vi "Provider_OnPopupMenu.vi"(11 "objects":T1[](array[typedef])) -> ()   [LabVIEW 2020, in "Actor Message Maker Provider.lvlib"]
uses:
  Actor Message Maker Provider.lvlib
  <resource>/Framework/Providers/API/mxLvMenuItem.ctl
  MessageMakerProvider/Support/Localized Strings.vi
  MessageMakerProvider/Message Maker Provider.lvlib
  MessageMakerProvider/AFPP Shared/Validation Mode.ctl
  MessageMakerProvider/AFPP Shared/AFPP Shared.lvlib
  <resource>/Framework/Providers/API/ItemRef.ctl
panel:
  out "error out":errorcluster
  in  "error in":errorcluster
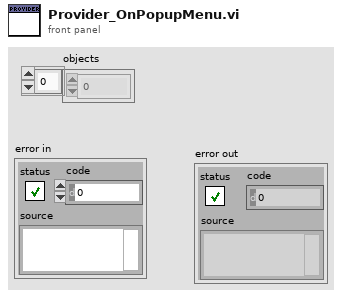
[diagram p1: front panel]
types:
  T1 = typedef "ItemRef.ctl" = u64
  T2 = typedef "AFPP Shared.lvlib/Validation Mode.ctl" = enum16{"An Actor Library", "A Target Tag"}
  T3 = typedef "mxLvMenuItem.ctl" = cluster{"Menu Name":string, "Description":string, "Icon File Name":path, "Menu Tag":string, "Enabled":bool, "Checked":bool, "Separator":bool, "Batchable":bool, "Weight":i32, "Batch Mode (Ignored if Not Batchable)":enum32{"Show If All Items Support Command", "Show If Any Items Support Command"}, "Menu Location":enum32{"<None>", "Project", "Project / Build Specifications", "Tools", "Tools / Source Control", "Tools / Real-Time Module", "Help"}, "Exclude From Getting Started Window Menu":bool}
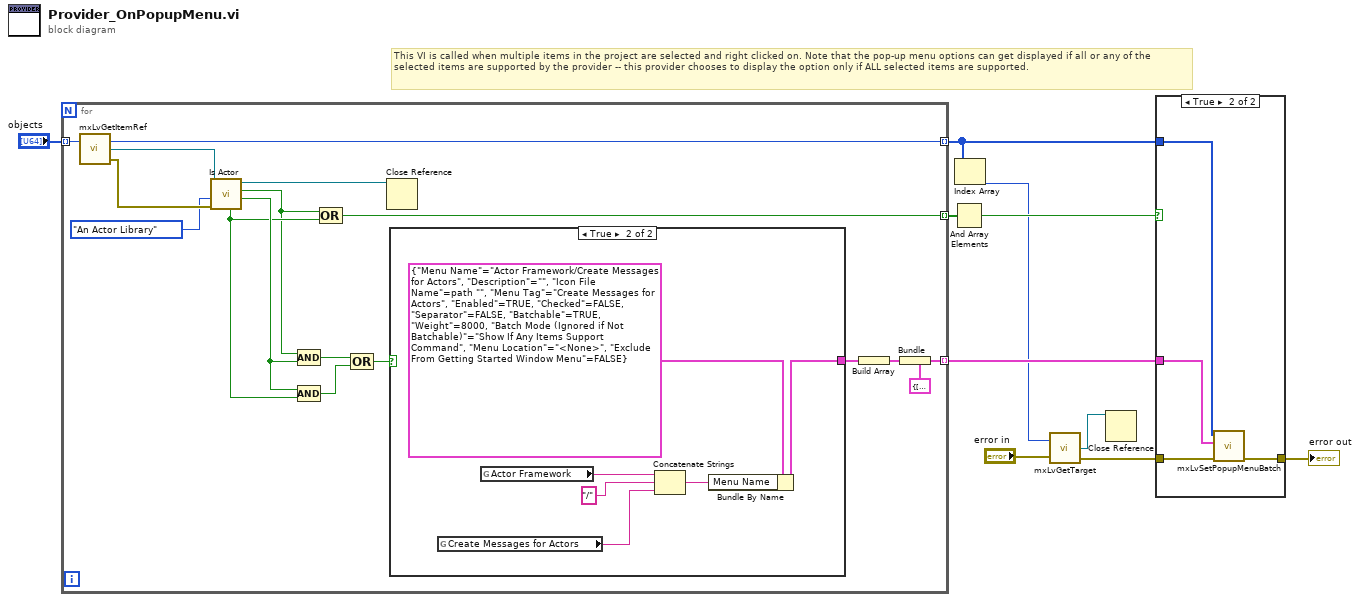
[diagram p0: block diagram]
diagram:
  # "This VI is called when multiple items in the project are selected and right clicked on. Note that the pop-up menu options can get displayed if all or any of the selected items are supported by the provider -- this provider chooses to display the option only if ALL selected items are supported."
  n1 = for {
    tunnel: [w27] -> w10 mode=indexing
    tunnel: "objects" -> [w26] mode=indexing
    tunnel: [w25] -> w2 mode=indexing
    tunnel: [w11] -> w7 mode=indexing
    n2 = call <resource>:"mxLvGetItemRef.vi"("Item"=w26) -> ("Item"=w25:T1, "Item Refnum"=w22:refnum<vi>, "error out"=w21:errorcluster)  [unwired: 1 in]
    n3 = call "Is Actor.vi"("error in (no error)"=w21, "Validation"=Validation_Mode."An Actor Library", "ProjectItem in"=w22) -> ("Has Public Methods"=w15:bool, "Is Actor"=w12:bool, "ProjectItem out"=w23:refnum<vi>, "Is Actor Interface"=w13:bool)  [unwired: 4 in, 1 out]
    n4 = Compound Arithmetic op=AND(w12, w15) -> (w16:bool)
    n5 = Compound Arithmetic op=AND(w15, w13) -> (w14:bool)
    n6 = Compound Arithmetic op=OR(w12, w13) -> (w11:bool)
    n7 = Compound Arithmetic op=OR(w16, w14) -> (w17:bool)
    n8 = Close Reference(reference=w23) -> ()  [unwired: 1 in, 1 out]
    n9 = case shown="True" w17 {
      tunnel: [_ w32] -> w20
      frame False {
      }
      frame True {
        n10 = global read "Localized Strings.vi" "Create Messages for Actors"() -> (w28:string)
        n11 = global read "Localized Strings.vi" "Actor Framework"() -> (w31:string)
        n12 = Concatenate Strings(w31, "/", w28) -> (w29:string)
        n13 = Bundle By Name(cluster=T3 {"Menu Name"="Actor Framework/Create Messages for Actors", "Description"="", "Icon File Name"=path "", "Menu Tag"="Create Messages for Actors", "Enabled"=TRUE, "Checked"=FALSE, "Separator"=FALSE, "Batchable"=TRUE, "Weight"=8000, "Batch Mode (Ignored if Not Batchable)"=enum."Show If Any Items Support Command", "Menu Location"=enum."<None>", "Exclude From Getting Started Window Menu"=FALSE} ("Menu Item"), "Menu Name"=w29) -> (w32:T3)
      }
    }
    n14 = Build Array(w20) -> (w19:T3[])
    n15 = Bundle(cluster=cluster{"Popup Menu Items":T3[]} {"Popup Menu Items"=[{"Menu Name"="", "Description"="", "Icon File Name"=path "", "Menu Tag"="", "Enabled"=TRUE, "Checked"=FALSE, "Separator"=FALSE, "Batchable"=TRUE, "Weight"=0, "Batch Mode (Ignored if Not Batchable)"=enum."Show If All Items Support Command", "Menu Location"=enum."<None>", "Exclude From Getting Started Window Menu"=FALSE}]}, "Popup Menu Items"=w19) -> (w27:cluster{"Popup Menu Items":T3[]})
  }
  n16 = And Array Elements(Boolean array=w7) -> (logical AND=w6:bool)
  n17 = Index Array(array=w2) -> (element=w1:T1)  [unwired: 1 in]
  n18 = call <resource>:"mxLvGetTarget.vi"("Item"=w1, "error in"="error in") -> ("Target"=w3:refnum<vi>, "error out"=w4:errorcluster)  [unwired: 1 out]
  n19 = Close Reference(reference=w3) -> ()  [unwired: 1 in, 1 out]
  n20 = case shown="True" w6 {
    tunnel: w10 -> [_ w38]
    tunnel: [w34 w37] -> w9
    tunnel: w4 -> [w34 w36]
    tunnel: w2 -> [_ w35]
    frame False {
    }
    frame True {
      n21 = call <resource>:"mxLvSetPopupMenuBatch.vi"("error in"=w36, "Menu Items"=w38, "Items"=w35) -> ("error out"=w37:errorcluster)  [unwired: 7 in, 1 out]
    }
  }
  "error out" <- w9
